vi "tetag.vi"(1 "Julian date at time of interest":dbl) -> (0 "Tetag (rad)":dbl)   [LabVIEW 2015]
panel:
  out "Tu":dbl
  out "GMST minuit":dbl
  out "Tetag0":dbl
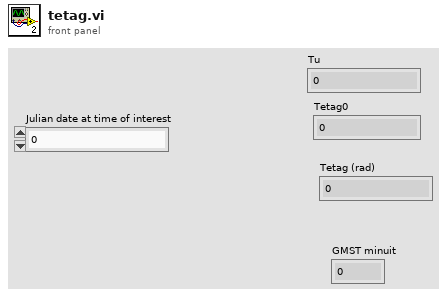
[diagram p1: front panel]
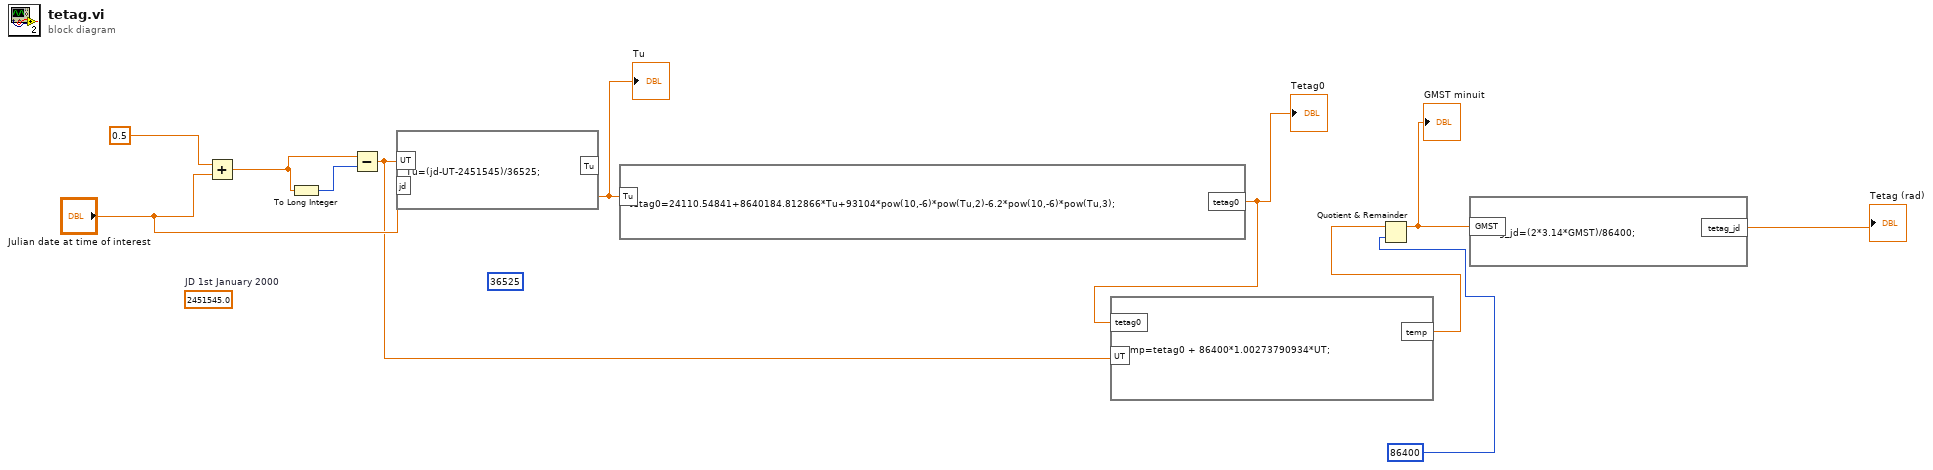
[diagram p0: block diagram]
diagram:
  (unwired) 36525
  (unwired) 2451545.0  # JD 1st January 2000
  n1 = Add(x=0.5, y="Julian date at time of interest") -> (x+y=w8:dbl)
  n2 = To Long Integer(number=w8) -> (32bit integer=w10:i32)
  n3 = Subtract(x=w8, y=w10) -> (x-y=w1:dbl)
  n4 = formula code="Tu=(jd-UT-2451545)/36525;"("UT"=w1, "jd"="Julian date at time of interest") -> ("Tu"=w2:dbl)
  "Tu" <- w2
  n5 = formula code="tetag0=24110.54841+8640184.812866*Tu+93104*pow(10,-6)*pow(Tu,2)-6.2*pow(10,-6)*pow(Tu,3);"("Tu"=w2) -> ("tetag0"=w6:dbl)
  "Tetag0" <- w6
  n6 = formula code="temp=tetag0 + 86400*1.00273790934*UT;"("tetag0"=w6, "UT"=w1) -> ("temp"=w5:dbl)
  n7 = Quotient & Remainder(x=w5, y=86400) -> (x-y*floor(x/y)=w11:dbl)  [unwired: 1 out]
  "GMST minuit" <- w11
  n8 = formula code="tetag_jd=(2*3.14*GMST)/86400;"("GMST"=w11) -> ("tetag_jd"=→"Tetag (rad)":dbl)
